vi "GetPublicKey.vi"(1 "e":cluster{"Boolean":bool, "Array":u64[]}, 2 "n":cluster{"Boolean":bool, "Array":u64[]}) -> (0 "Public Key":string)   [LabVIEW 2023]
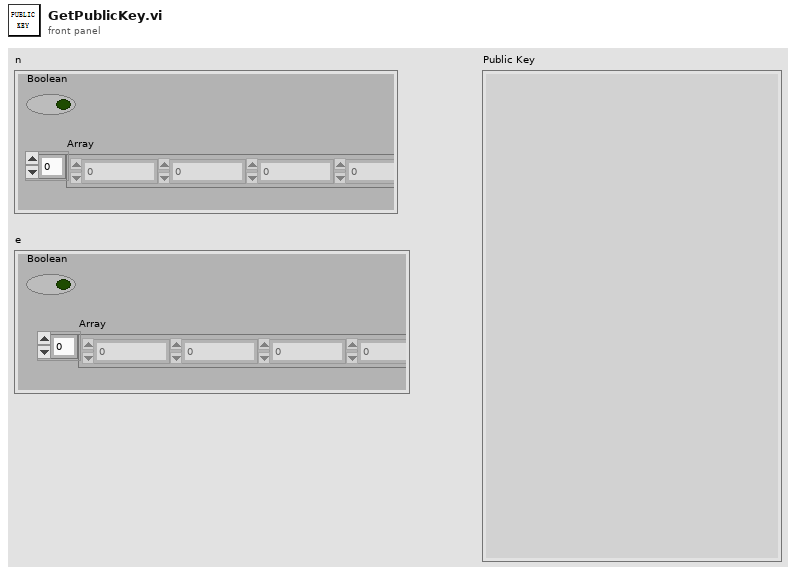
[diagram p1: front panel]
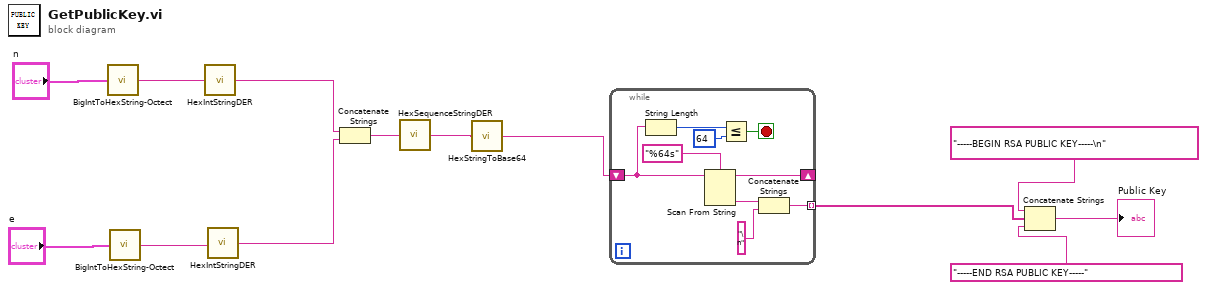
[diagram p0: block diagram]
diagram:
  n1 = call "BigIntToHexString-Octect.vi"("a"="n") -> ("Hex string"=w13:string)
  n2 = call "BigIntToHexString-Octect.vi"("a"="e") -> ("Hex string"=w12:string)
  n3 = call "HexIntStringDER.vi"("Hex(formatted integer)"=w13) -> ("DER"=w11:string)
  n4 = call "HexIntStringDER.vi"("Hex(formatted integer)"=w12) -> ("DER"=w10:string)
  n5 = Concatenate Strings(w11, w10) -> (w9:string)
  n6 = call "HexSequenceStringDER.vi"("Hex(sequence)"=w9) -> ("DER"=w4:string)
  n7 = call "HexStringToBase64.vi"("Hex"=w4) -> ("BASE64 string"=w3:string)
  n8 = while {
    shift-right: [w22] -> _
    shift-left: w3 -> [w17]
    tunnel: [w18] -> w8 mode=indexing
    stop <- w14 stop-if-true
    n9 = String Length(string=w17) -> (length=w16:i32)
    n10 = Scan From String(format string="%64s", input string=w17) -> (remaining string=w22:string, output 1=w19:string)  [unwired: 3 in, 2 out]
    n11 = Less Or Equal?(x=w16, y=64) -> (x <= y?=w14:bool)
    n12 = Concatenate Strings(w19, "\n") -> (w18:string)
  }
  n13 = Concatenate Strings("-----BEGIN RSA PUBLIC KEY-----\n", w8, "-----END RSA PUBLIC KEY-----") -> (→"Public Key":string)
